vi "Read Sub panel M.vi"(8 "error in (no error)":errorcluster, 11 "Actor M in":refnum<class "Actor M.lvclass">) -> (0 "error out":errorcluster, 2 "Sub panel M":refnum<vi>, 3 "Actor M out":refnum<class "Actor M.lvclass">)   [LabVIEW 2019, in "Actor M.lvlib" / "Actor M.lvclass"]
uses:
  Actor M.lvclass
  Actor M.lvclass/Actor M.ctl
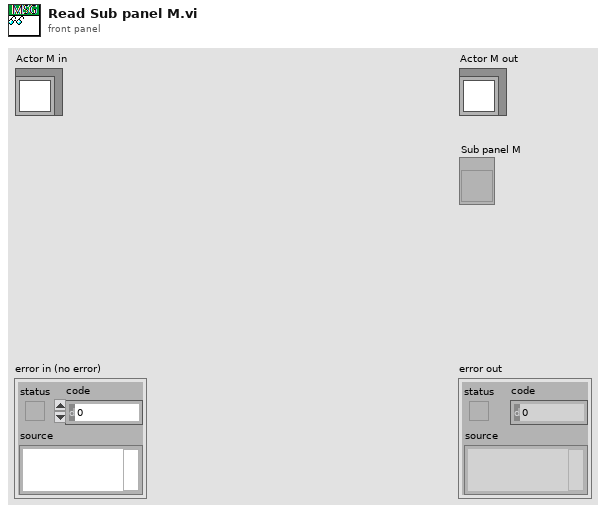
[diagram p1: front panel]
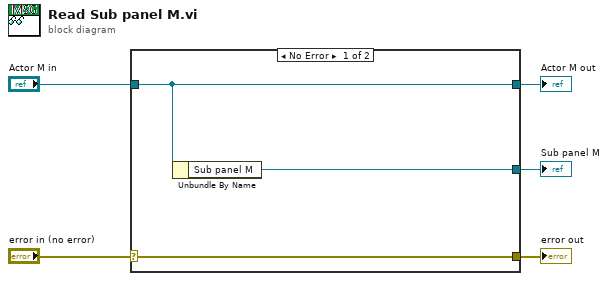
[diagram p0: block diagram]
diagram:
  n1 = case shown="No Error" "error in (no error)" {
    selector: "error in (no error)" -> [w8 w9]
    tunnel: [w8 w9] -> w4
    tunnel: [w7 w10] -> w2
    tunnel: "Actor M in" -> [w7 w10]
    tunnel: [w6 _] -> w1
    frame No Error {
      n2 = Unbundle By Name(w7) -> ("Sub panel M"=w6:refnum<vi>)
    }
    frame Error {
    }
  }
  "error out" <- w4
  "Actor M out" <- w2
  "Sub panel M" <- w1
